vi "DVR_Timer.vi"(7 "Action":enum16{"Create", "Start", "Get", "Destroy"}(ring), 8 "error in (no error)":errorcluster) -> (0 "error out":errorcluster, 2 "ElapsedTime":u32)   [LabVIEW 2018]
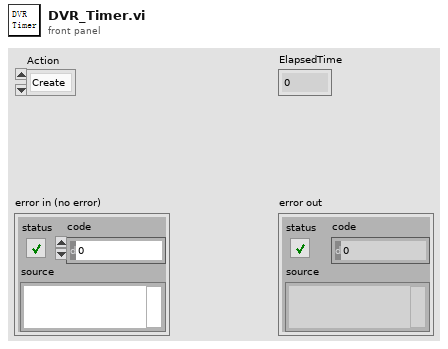
[diagram p1: front panel]
types:
  T1 = cluster{"Start Time":u32, "Elapsed Time":u32, "Running?":bool}
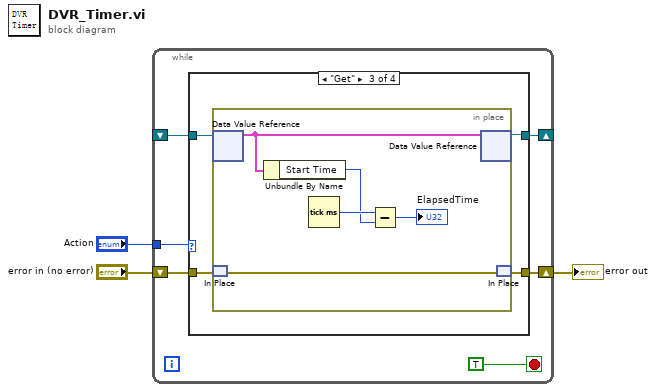
[diagram p0: block diagram]
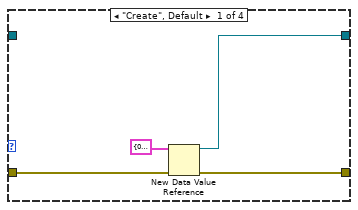
[diagram p2: hidden frame]
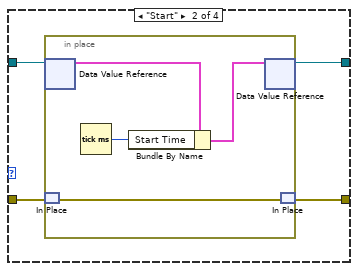
[diagram p3: hidden frame]
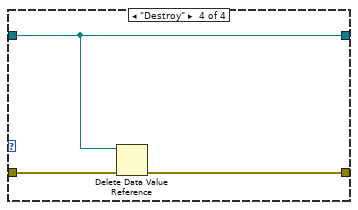
[diagram p4: hidden frame]
diagram:
  n1 = while {
    tunnel: "Action" -> [w8]
    shift-right: [w5] -> _
    shift-left: _ -> [w4]
    shift-right: [w6] -> w1
    shift-left: "error in (no error)" -> [w7]
    stop <- TRUE stop-if-true
    n2 = case shown="\"Get\"" w8 {
      tunnel: w7 -> [w12 w17 w25 w33]
      tunnel: [w11 w16 w24 w32] -> w6
      tunnel: [w10 w14 w22 w31] -> w5
      tunnel: w4 -> [_ w15 w23 w31]
      frame "Create", Default {
        n3 = New Data Value Reference(data value=T1 {"Start Time"=0, "Elapsed Time"=0, "Running?"=TRUE}, error in=w12) -> (data value reference=w10:refnum<data-value>, error out=w11:errorcluster)
      }
      frame "Start" {
        n4 = in-place {
          n5 = in-place-dvr #1(w15) -> (w20:T1)  [unwired: 1 out]
          n6 = in-place-match #2(w17) -> (w21:errorcluster)
          n7 = Tick Count (ms)() -> (millisecond timer value=w19:u32)
          n8 = Bundle By Name(cluster=w20, "Start Time"=w19) -> (w18:T1)
          n9 = in-place-dvr #1(w18) -> (w14:refnum<data-value>)  [unwired: 1 out]
          n10 = in-place-match #2(w21) -> (w16:errorcluster)
        }
      }
      frame "Get" {
        n11 = in-place {
          n12 = in-place-dvr #3(w23) -> (w28:T1)  [unwired: 1 out]
          n13 = in-place-match #4(w25) -> (w30:errorcluster)
          n14 = Unbundle By Name(w28) -> ("Start Time"=w27:u32)
          n15 = Tick Count (ms)() -> (millisecond timer value=w29:u32)
          n16 = Subtract(x=w29, y=w27) -> (x-y=→"ElapsedTime":u32)
          n17 = in-place-dvr #3(w28) -> (w22:refnum<data-value>)  [unwired: 1 out]
          n18 = in-place-match #4(w30) -> (w24:errorcluster)
        }
      }
      frame "Destroy" {
        n19 = Delete Data Value Reference(data value reference=w31, error in=w33) -> (error out=w32:errorcluster)  [unwired: 1 out]
      }
    }
  }
  "error out" <- w1
